vi "LoadScreenInHmiScheduler.vi"(7 "Enum Screen":T1, 8 "error in (no error)":errorcluster) -> (0 "error out":errorcluster)   [LabVIEW 2013]
uses:
  enumScreen.ctl
  030 - EVENTS/EnumFgvEventCommand.ctl
  030 - EVENTS/01 - ToHmiScheduler/ToHmiScheduler.ctl
  030 - EVENTS/01 - ToHmiScheduler/ToHmiSchedulerCommand.ctl
  030 - EVENTS/03 - ToMessageHandlerProcess/ToMessageHandlerEvent.ctl
  030 - EVENTS/03 - ToMessageHandlerProcess/enumMessageCriticity.ctl
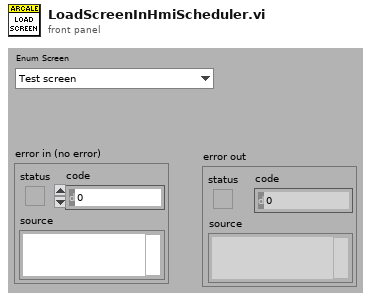
[diagram p1: front panel]
types:
  T1 = typedef "enumScreen.ctl" = enum16{"Test screen", "Ecran principal", "LOG", "Setup", "Popup : About", "Popup : View last message", "Popup : WebBrowser help", "Traduction", "Popup : DEBUG Process"}
  T2 = typedef "ToHmiSchedulerCommand.ctl" = enum16{"Load screen", "Lock screen", "Unlock screen", "Close enable", "Close disable", "Start automatic progress bar", "Stop automatic progress bar", "Set progress bar value (0..100)", "Load previous screen", "Close application", "View message", "Clear message", "Set Window State"}
  T3 = typedef "ToHmiScheduler.ctl" = cluster{"Command":T2, "Screen path":path, "Progress bar value":u8, "Screen Title":string, "To message handler event":T4, "Window_State":enum32{"Invalid", "Standard", "Closed", "Hidden", "Minimized", "Maximized"}}
  T4 = typedef "ToMessageHandlerEvent.ctl" = cluster{"date / time":timestamp, "Criticity":T5, "Emitter":string, "Message":string}
  T5 = typedef "enumMessageCriticity.ctl" = enum16{"No error", "Info", "Warning", "Error", "Fatal error"}
  T6 = typedef "EnumFgvEventCommand.ctl" = enum16{"Setup", "Cleanup", "Get"}
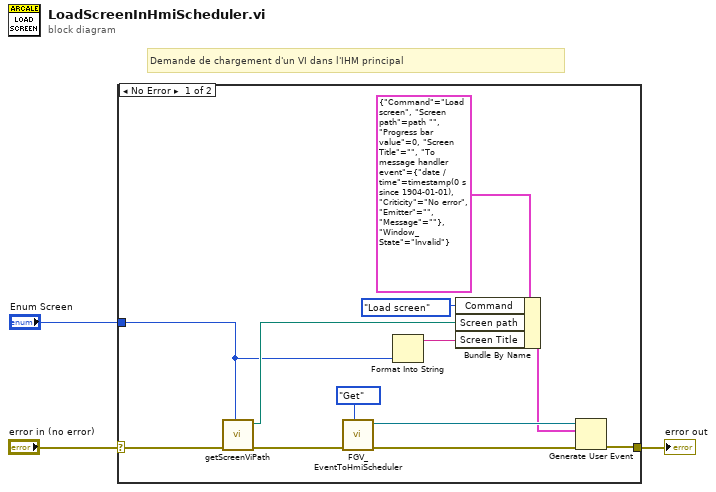
[diagram p0: block diagram]
diagram:
  # "Demande de chargement d'un VI dans l'IHM principal"
  n1 = case shown="No Error" "error in (no error)" {
    selector: "error in (no error)" -> [w15 w16]
    tunnel: "Enum Screen" -> [w5 _]
    tunnel: [w6 w16] -> w1
    frame No Error {
      n2 = call "getScreenViPath.vi"("Enum Screen"=w5, "error in (no error)"=w15) -> ("error out"=w14:errorcluster, "Path"=w7:path)  [unwired: 8 in]
      n3 = call "FGV_EventToHmiScheduler.vi"("Command"=EnumFgvEventCommand."Get", "error in (no error)"=w14) -> ("error out"=w12:errorcluster, "ToHmiSchedulerEvent"=w11:refnum<user-event>)  [unwired: 8 in]
      n4 = Format Into String(w5) -> (resulting string=w4:string)  [unwired: 3 in, 1 out]
      n5 = Bundle By Name(cluster=T3 {"Command"=enum."Load screen", "Screen path"=path "", "Progress bar value"=0, "Screen Title"="", "To message handler event"={"date / time"=timestamp(0 s since 1904-01-01), "Criticity"=enum."No error", "Emitter"="", "Message"=""}, "Window_State"=enum."Invalid"} ("event data"), "Command"=ToHmiSchedulerCommand."Load screen", "Screen path"=w7, "Screen Title"=w4) -> (w9:T3)
      n6 = Generate User Event(user event=w11, event data cluster=w9, error in=w12) -> (error out=w6:errorcluster)  [unwired: 1 in, 1 out]
    }
    frame Error {
    }
  }
  "error out" <- w1
